vi "HardWare_Phsical Channels Config_Gantner.vi"() -> ()   [LabVIEW 2016]
uses:
  ToolKit/Popup/Public/PSPOP_Popup Cluster.ctl
  ToolKit/Popup/Private/Ctrls/PSPOP_Grid.Cell Info.ctl
  ToolKit/Popup/Private/Ctrls/POP_Data Type.ctl
  HardWare/Ctrls/HardWare _ Data Queue Manage FGV Operation.ctl
  ToolKit/Toolbar/net/SubVIs/TBA_NET_Item.ctl
  HardWare/Ctrls/HardWare Gen _ DAQ Queue Names FGV Operations.ctl
  HardWare/Gantner/DAQ FGV Operations.ctl
  Architecture/Queue Management/ARC_Queue Create_Single.vi
  Architecture/Queue Management/ARC_Queue Remove Element.vi
  Architecture/Queue Management/ARC_Queue Valid.vi
  Architecture/Queue Management/ARC_Queue Insert Element.vi
  Architecture/Queue Management/ARC_Queue Destroy_Single.vi
panel:
  in  "Popups":T1 {"Time" format="%<%Y/%m/%d %I:%M:%S>T"; "Boolean" items=["False", "True"]; "Ring" items=["False", "True"]}
  in  "Cell Info (type only)":T2={"Tag"="", "Row"=0, "Column"=0, "In Symbol?"=FALSE, "In Data?"=FALSE, "Cell String"="", "Ctl Refnum"=refnum, "Prop Type"=enum."Unkown", "Ring Strings"=[], "Ring Values"=[], "New Cell String"=""}
  in  "Tree":string(tree)
  out "Current State":string
  in  "Parameter":cluster{"Q-Local":string, "Variant":variant}
  # "/* -------- Notes for All Users -------- */\nRecommand : \n[1].Display Setting Resolution -> 1440x900\n[2].Read Arch Notes First.\n[3].Make A Call When You Are In Trouble.\n\nTeam Members:\nPansino Soft,Pansino SDMA\n\nCopyright@2013 Pansino.Beijing\n\nVersion Number: 2013"
  # "Boolean Colors"
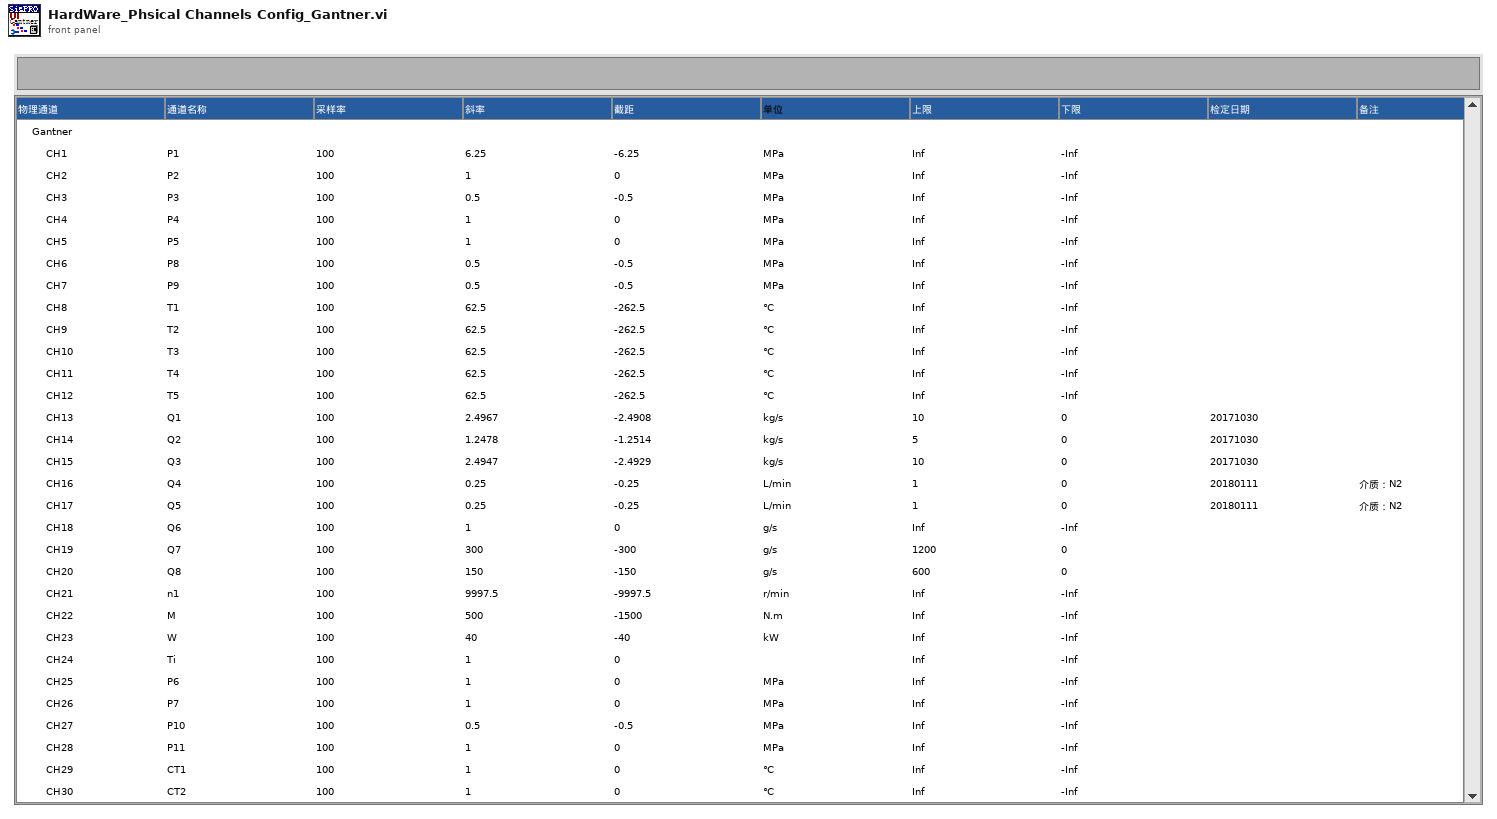
[diagram p1: front panel]
types:
  T1 = typedef "PSPOP_Popup Cluster.ctl" = cluster{"Unknown":bool, "Unknown 2":bool, "String":string, "Integer":i32, "Float":dbl, "Color":u32, "Boolean":u32, "Ring":u32, "Captioned String":cluster{"String":string, "OK":bool, "Cancel":bool}, "Captioned Integer":cluster{"First":i32, "OK":bool, "Cancel":bool}, "Boolean Colors":cluster{"False":cluster{"FG":u32, "BG":u32}, "True":cluster{"FG":u32, "BG":u32}, "T  to  F":cluster{"FG":u32, "BG":u32}, "F  to  T":cluster{"FG":u32, "BG":u32}, "OK":bool, "Cancel":bool}, "2-Int Cluster":cluster{"First":i32, "Second":i32, "OK":bool, "Cancel":bool}, "4-Int Cluster":cluster{"First":i32, "Second":i32, "Third":i32, "Fourth":i32, "OK":bool, "Cancel":bool}, "6-Dbl Cluster":cluster{"First":dbl, "Second":dbl, "Third":dbl, "Fourth":dbl, "Fourth 2":dbl, "Third 2":dbl, "OK":bool, "Cancel":bool}, "Path":path, "Combox":string, "Time":timestamp, "ShortCut":string}
  T2 = typedef "PSPOP_Grid.Cell Info.ctl" = cluster{"Tag":string, "Row":i32, "Column":i32, "In Symbol?":bool, "In Data?":bool, "Cell String":string, "Ctl Refnum":refnum<vi>, "Prop Type":T3, "Ring Strings":string[], "Ring Values":ext[], "New Cell String":string}
  T3 = typedef "POP_Data Type.ctl" = enum16{"NO POPUP", "Unkown", "String", "Integer", "Float", "Color", "Boolean", "Ring", "Captioned String", "Captioned Integer", "Button Color", "2 Int Cluster", "4 Int Cluster", "6-Dbl Cluster", "Path", "Combox", "Time", "ShotCut String"}
  T4 = cluster{"LocalName":string, "System Config":path, "DynaThreads":path, "DataBuf":refnum<queue>, "VIRef":refnum<vi>}
  T5 = typedef "HardWare _ Channel Configurations PopUp Type.ctl" = cluster{"Pop Type":T3, "PopValue":string}
  T6 = cluster{"Error":errorcluster, "Ref":cluster{"VIRef":refnum<vi>, "Tree":refnum<vi>, "CallerVI":refnum<vi>}, "Exit":bool, " Paths":cluster{"PathInActive":path, "ModCfg":path, "CHdef":path, "DT folder":path}, "Q-Local":cluster{"Q-Local Name":string, "Q-Local Order":string, "Q-Local Data":variant}, "Q-HighLevel":cluster{"Q-HighLevel Name":string, "Q-HighLevel Order":string, "Q-HighLevel Data":variant}, "Q-DAQ":cluster{"Q-LowLevel Name[]":string[], "Q-LowLevel Order":string, "Q-LowLevel Data":variant}, "PopUp":string, "Chan Para":cluster{"ParaNames":string[], "DfltValues":string[], "Types":string[], "PopTypes":T5[]}, "Q_DAQs[]":string[], "ActiveModu":cluster{"Tag":string, "CHtype":string}, "ColInfo":cluster{"ColName[]":string[], "ColAlias[]":string[], "ColLength[]":i32[]}, "UsedChList[]":cluster{"ModuTag":string, "ModuAlias":string, "ChanTag[]":string[], "ChanAlias[]":string[], "ChanUnit[]":string[]}[], "DataBuf":refnum<queue>, "Units[]":string[], "ColHeaders[]":string[]}
  T7 = typedef "HardWare _ Data Queue Manage FGV Operation.ctl" = enum16{"Initialize", "Add", "Read", "All"}
  T8 = typedef "TBA_NET_Item.ctl" = cluster{"Tag":string, "Name":string, "Tip":string, "Image":path, "DisplayStyle":i32, "Enable":bool, "Visible":bool}
  T9 = cluster{"Status":string[], "Item":cluster{"Item":T8[]}[]}
  T10 = typedef "HardWare Gen _ DAQ Queue Names FGV Operations.ctl" = enum16{"Initialize", "AddName", "ReadName"}
  T11 = cluster{"Column":i32, "Row":i32, "Formula":string}
  T12 = typedef "DAQ FGV Operations.ctl" = enum16{"Search", "ReadCFG", "ReadVCH", "UpdateTempCFG", "DownloadCFG", "OpenCFG", "ImportPara", "Config", "Start", "Read", "Stop", "Clear"}
  T13 = cluster{"ParaNames":string[], "DfltValues":string[], "Types":string[], "PopTypes":T5[]}
  T14 = cluster{"Q-Local Name":string, "输出簇 2":cluster{"Status":string[], "Item":cluster{"Item":T8[]}[]}}
  T15 = cluster{"Q-Local Name":string, "DataBuf":refnum<queue>}
  T16 = cluster{"ModuTag":string, "ModuAlias":string, "ChanTag[]":string[], "ChanAlias[]":string[], "ChanUnit[]":string[]}[]
  T17 = cluster{"ParaNames":string[], "DfltPara":string[], "Types":string[], "PopTypes":T5[]}
  T18 = cluster{"ColName[]":string[], "ColAlias[]":string[], "ColLength[]":i32[]}
  T19 = typedef "HardWare _ Module Configuration.ctl" = cluster{"ModuName":string, "ModuAlias":string, "ModuSN":string, "CHtype":string, "ParaNames[]":string[], "Paravalues[]":string[][]}
  T20 = cluster{"SlopeA":string, "InterceptB":string, "Unit":string, "AlarmMax":string, "AlarmMin":string, "CheckTime":string, "Note":string, "ChanName":string, "SensorNo.":string}[]
  T21 = typedef "LVPoint32TypeDef.ctl" = cluster{"Horizontal":i32, "Vertical":i32}
  T22 = typedef "POP_Popup Call Parameters.ctl" = cluster{"Prop Type":T3, "Initial Value":variant, "Caption Strings":string[], "Ring Strings":string[], "Cell Rect":cluster{"left":i16, "top":i16, "right":i16, "bottom":i16}, "Mouse Coords":cluster{"x":i16, "y":i16}, "Call Data":variant, "Ring Values":ext[], "Browse Options":T23, "Combo Box":cluster{"Allow Undefined Strings":bool}}
  T23 = typedef "LVBrowseOptionsTypeDef.ctl" = cluster{"Prompt":string, "Match Pattern":string, "Mode":enum32{"existing file", "new file", "new or existing file", "existing dir", "new dir", "new or existing dir", "existing file (use LLBs)", "new file (use LLBs)", "new or existing file (use LLBs)", "new or existing file or directory (use LLBs)", "existing dir (use LLBs)", "new dir (use LLBs)", "new or existing dir (use LLBs)", "existing file or dir", "new file or dir", "new or existing file or dir", "existing file or dir (use LLBs)", "new file or dir (use LLBs)"}, "Start Path":path, "Pattern Label":string, "Button Text":string}
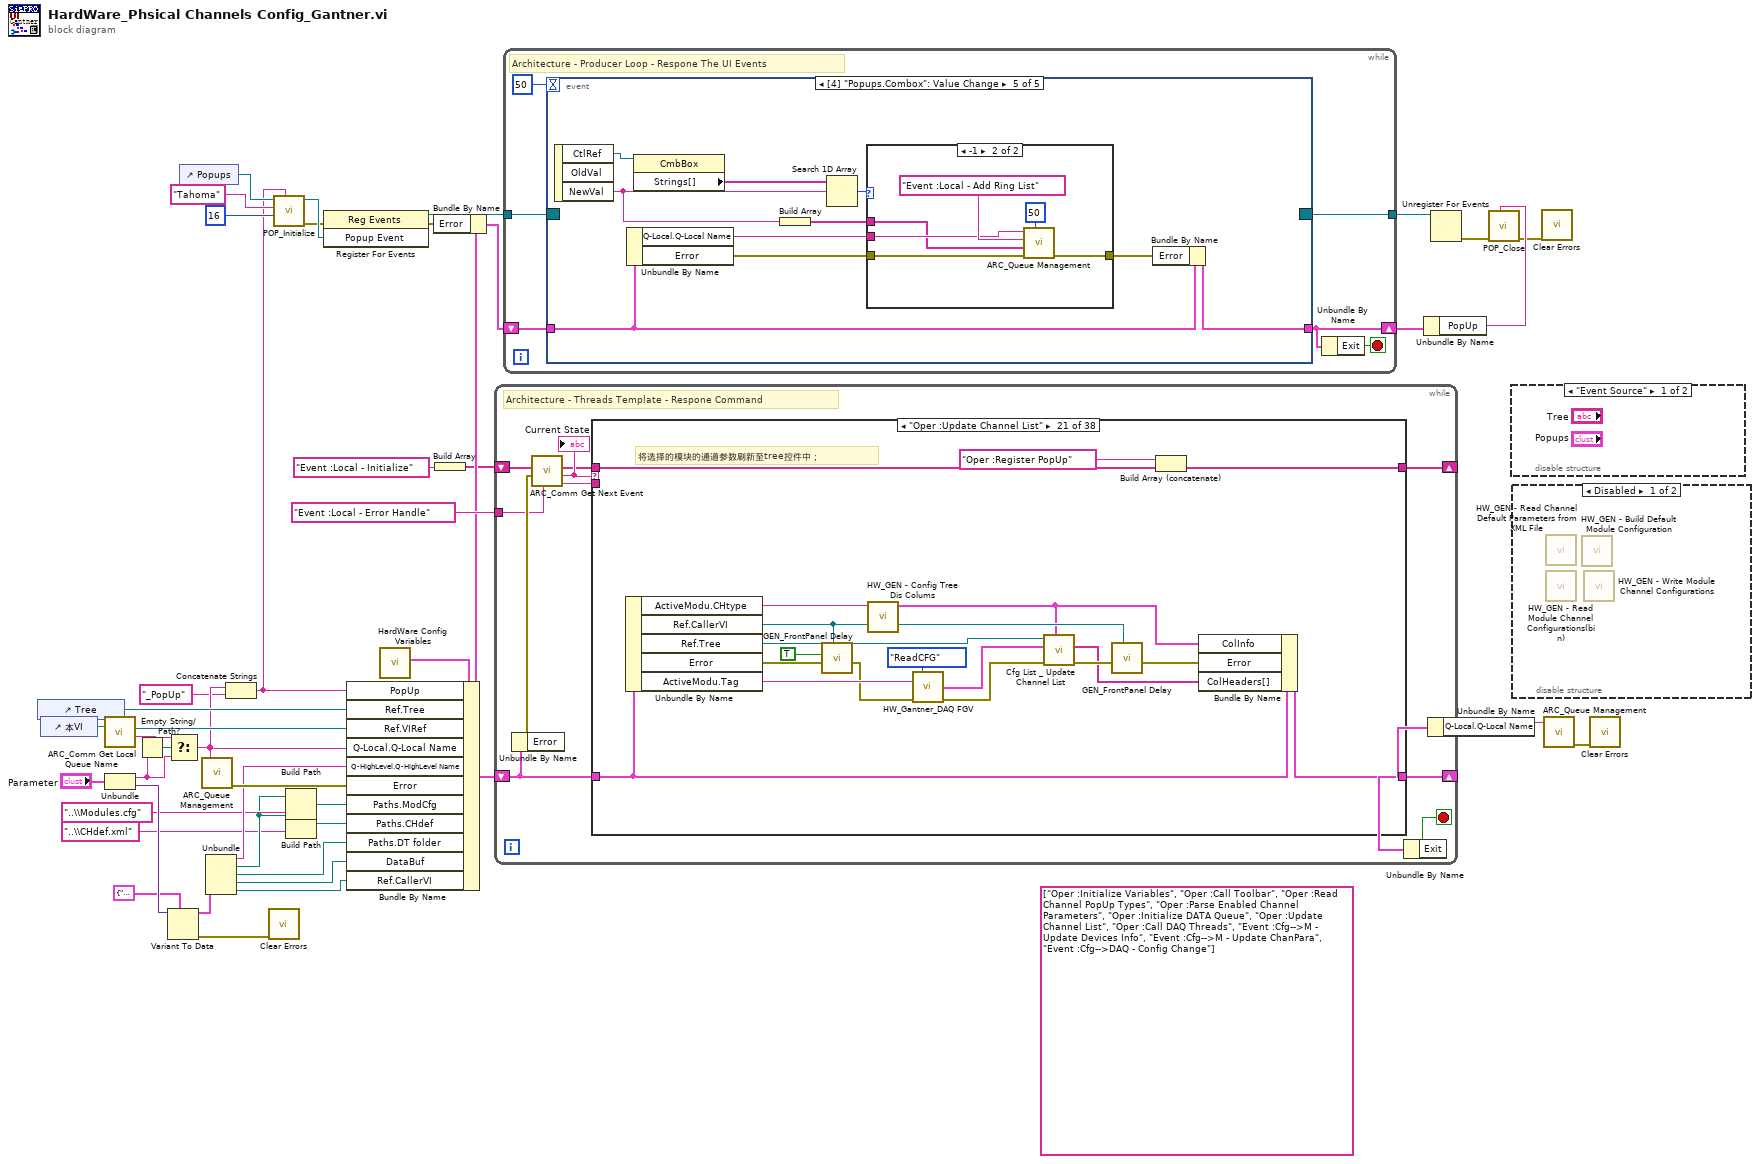
[diagram p0: block diagram]
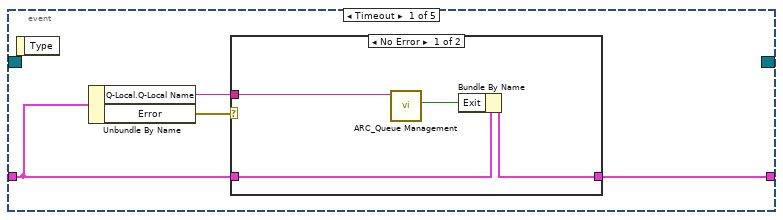
[diagram p3: hidden frame]
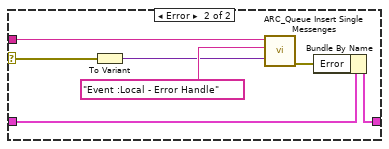
[diagram p4: hidden frame]
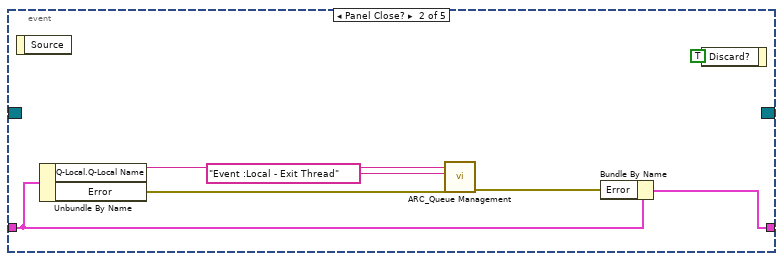
[diagram p5: hidden frame]
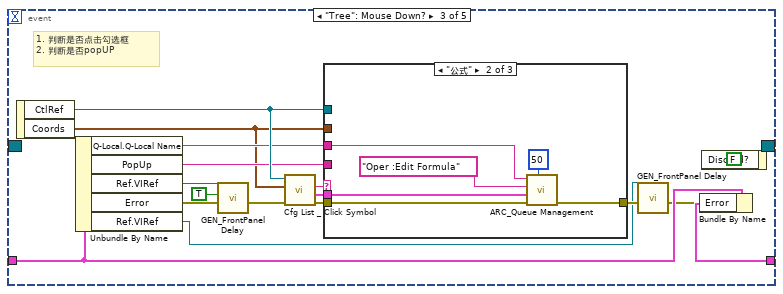
[diagram p6: hidden frame]
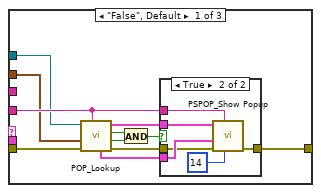
[diagram p7: hidden frame]
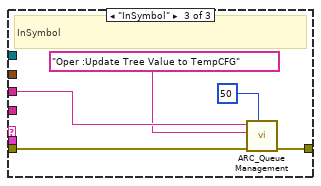
[diagram p9: hidden frame]
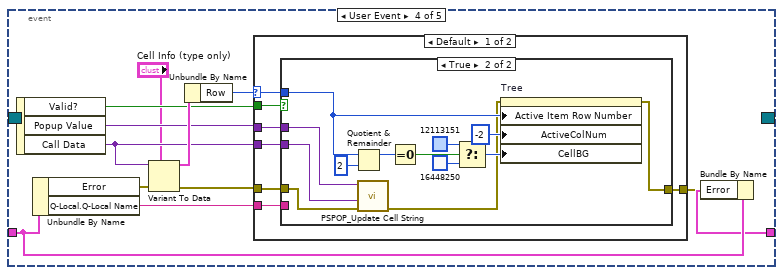
[diagram p10: hidden frame]
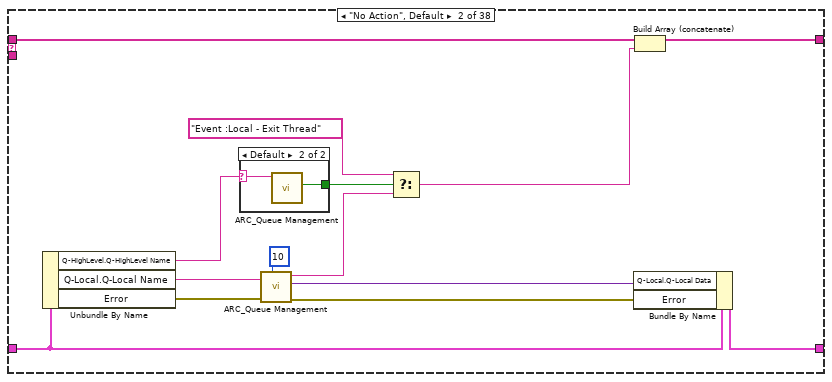
[diagram p16: hidden frame]
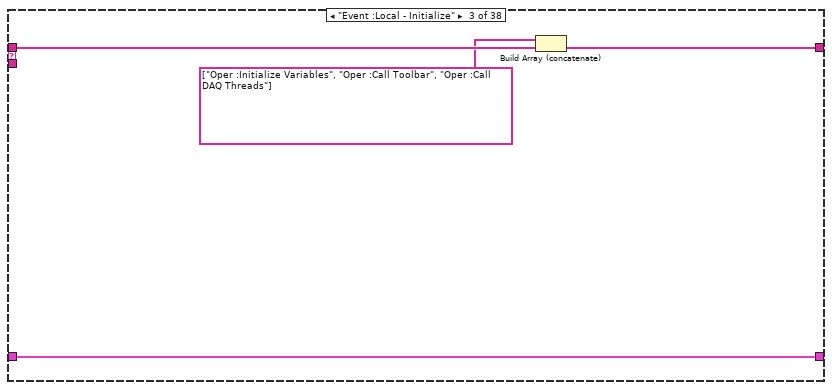
[diagram p18: hidden frame]
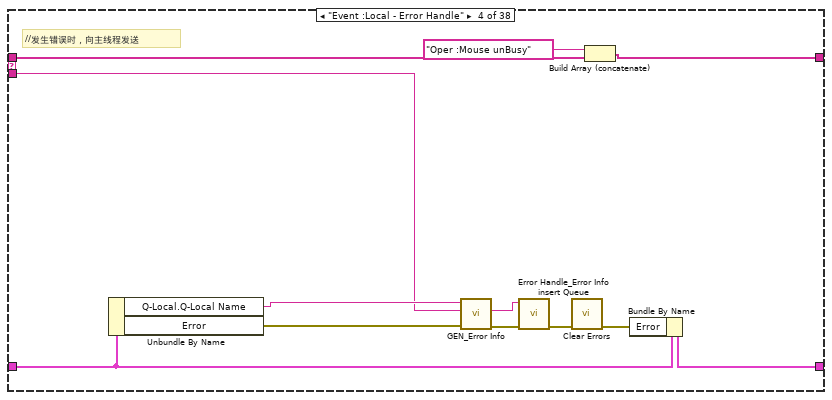
[diagram p19: hidden frame]
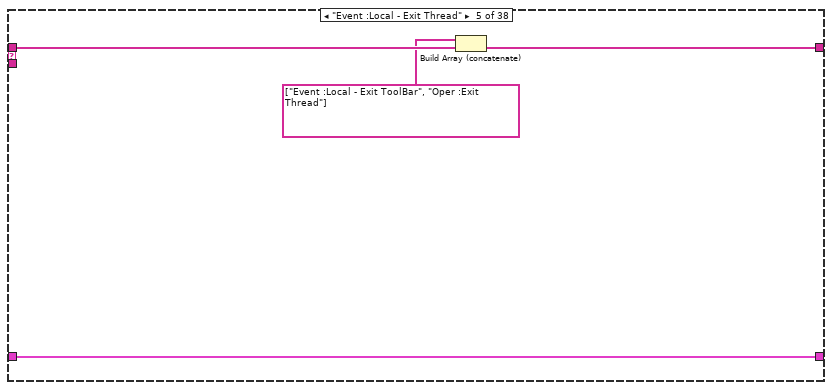
[diagram p20: hidden frame]
diagram:
  (unwired) string[] ["Oper :Initialize Variables", "Oper :Call Toolbar", "Oper :Read Channel PopUp Types", "Oper :Parse Enabled Channel Parameters", "Oper :Initialize DATA Queue", "Oper :Update Channel List", "Oper :Call DAQ Threads", "Event :Cfg-->M - Update Devices Info", "Event :Cfg-->M - Update ChanPara", "Event :Cfg-->DAQ - Config Change"] ("数组")
  n1 = control-ref of="Tree"() -> (w28:refnum<vi>)
  n2 = control-ref of="本VI"() -> (w30:refnum<vi>)
  n3 = call "ARC_Comm Get Local Queue Name.vi"("VI Ref"=w30) -> ("VI  Name"=w31:string, "VI Ref out"=w29:refnum<vi>)  [unwired: 8 in, 1 out]
  n4 = Unbundle("Parameter") -> ("Q-Local"=w33:string, "Variant"=w43:variant)
  n5 = Empty String/Path?(string/path=w33) -> (empty?=w34:bool)
  n6 = Variant To Data(type=T4 {"LocalName"="", "System Config"=path "", "DynaThreads"=path "", "DataBuf"=refnum, "VIRef"=refnum} ("output cluster"), Variant=w43) -> (data=w44:T4, error out=w35:errorcluster)  [unwired: 1 in]
  n7 = Select(t=w31, s=w34, f=w33) -> (s? t:f=w22:string)
  n8 = control-ref of="Popups"() -> (w27:refnum<vi>)
  n9 = call-poly "ARC_Queue Management.vi"("Queue Name"=w22) -> ("error out"=w45:errorcluster)  [unwired: 8 in, 2 out]
  n10 = Unbundle(w44) -> ("LocalName"=w11:string, "System Config"=w6:path, "DynaThreads"=w10:path, "DataBuf"=w3:refnum<queue>, "VIRef"=w1:refnum<vi>)
  n11 = Concatenate Strings(w22, "_PopUp" ("字符串")) -> (w12:string)
  n12 = call <vilib>:"Clear Errors.vi"("error in (no error)"=w35) -> ()  [unwired: 5 in, 2 out]
  n13 = call "POP_Initialize.vi"("Name"=w12, "Font Size"=u32 16, "TontName"="Tahoma", "Popup Cluster Ref"=w27) -> ("error out"=w23:errorcluster, "Popup Event"=w24:refnum<user-event>)  [unwired: 6 in]
  n14 = Build Path(base path=w6, name or relative path="..\\Modules.cfg" ("名称或相对路径")) -> (appended path=w9:path)
  n15 = Build Path(base path=w6, name or relative path="..\\CHdef.xml" ("名称或相对路径")) -> (appended path=w7:path)
  n16 = register-events(error in=w23, w24) -> (reference out=w20:refnum<event-registration>, error out=w18:errorcluster)  [unwired: 1 in]
  n17 = call "HardWare Config Variables.vi"() -> ("HardWare_Phsical Channels Config.vi"=w32:T6)  [unwired: 11 in]
  n18 = Bundle By Name(cluster=w32, "PopUp"=w12, "Ref.Tree"=w28, "Ref.VIRef"=w29, "Q-Local.Q-Local Name"=w22, "Q-HighLevel.Q-HighLevel Name"=w11, "Error"=w45, "Paths.ModCfg"=w9, "Paths.CHdef"=w7, "Paths.DT folder"=w10, "DataBuf"=w3, "Ref.CallerVI"=w1) -> (w38:T6)
  n19 = Bundle By Name(cluster=w38, "Error"=w18) -> (w19:T6)
  n20 = Build Array("Event :Local - Initialize") -> (w36:string[])
  n21 = while {
    shift-right: [w49] -> w41
    shift-left: w38 -> [w51]
    shift-right: [w52] -> _
    shift-left: w36 -> [w55]
    tunnel: "Event :Local - Error Handle" ("Error Handle") -> [w47]
    stop <- w48 stop-if-true
    # "Architecture - Threads Template - Respone Command"
    n22 = Unbundle By Name(w51) -> ("Error"=w50:errorcluster)
    n23 = call "ARC_Comm Get Next Event.vi"("Error Handle"=w47, "error in (no error)"=w50, "event queue in"=w55) -> ("prev event"=w46:string, "next event"=w54:string, "event queue out"=w53:string[])  [unwired: 3 in]
    "Current State" <- w54
    n24 = case shown="\"Oper :Update Channel List\"" w54 {
      selector: w54 -> [_ _ _ _ _ _ _ _ _ _ _ _ _ _ _ _ _ _ _ _ _ _ _ _ _ _ _ _ _ _ _ _ w420 w426 w432 _ _ _]
      tunnel: w51 -> [w56 w71 w76 w87 w90 w100 w107 w111 w123 w134 w154 w178 w181 w201 w213 w217 w220 w225 w229 w236 w256 w261 w271 w280 w284 w303 w316 w332 w367 w402 w413 w416 w419 w425 w431 w437 w444 w459]
      tunnel: w53 -> [w57 w69 w77 w89 w93 w101 w104 w112 w124 w135 w155 w179 w197 w200 w210 w218 w223 w228 w230 w238 w257 w269 w273 w281 w283 w288 w317 w337 w363 w403 w415 w417 w424 w430 w436 w438 w447 w462]
      tunnel: [w57 w68 w75 w85 w92 w98 w109 w112 w124 w135 w153 w177 w197 w199 w209 w215 w223 w228 w230 w238 w248 w269 w272 w281 w285 w287 w315 w337 w362 w390 w414 w417 w423 w429 w435 w438 w447 w462] -> w52
      tunnel: [w56 w70 w76 w88 w90 w99 w110 w111 w120 w133 w142 w176 w180 w201 w212 w216 w220 w225 w229 w234 w253 w260 w270 w280 w284 w292 w316 w331 w366 w392 w413 w416 w421 w427 w433 w437 w443 w458] -> w49
      tunnel: w46 -> [_ _ _ w79 _ _ _ _ _ _ _ _ _ _ _ _ _ _ _ _ _ _ _ _ _ _ _ _ _ w395 _ _ _ _ _ _ _ _]
      frame "----------Core Status----------" {
      }
      frame "No Action", Default {
        n25 = Unbundle By Name(w71) -> ("Q-HighLevel.Q-HighLevel Name"=w63:string, "Q-Local.Q-Local Name"=w64:string, "Error"=w65:errorcluster)
        n26 = case shown="Default" w63 {
          selector: w63 -> [_ w72]
          tunnel: [_ w73] -> w61
          frame "" {
          }
          frame Default {
            n27 = call-poly "ARC_Queue Management.vi"("Queue Name(unamed)"=w72) -> ("Not Exist?"=w73:bool)  [unwired: 8 in, 2 out]
          }
        }
        n28 = call-poly "ARC_Queue Management.vi"("Time out(-1)_queue out"=10, "error in (no error)"=w65, "Queue Name(unamed)"=w64) -> ("error out"=w67:errorcluster, "Data"=w66:variant, "Event"=w59:string)  [unwired: 5 in, 1 out]
        n29 = Select(t="Event :Local - Exit Thread" ("Event"), s=w61, f=w59) -> (s? t:f=w58:string)
        n30 = Bundle By Name(cluster=w71, "Q-Local.Q-Local Data"=w66, "Error"=w67) -> (w70:T6)
        n31 = Build Array (concatenate)(w69, w58) -> (w68:string[])
      }
      frame "Event :Local - Initialize" {
        n32 = Build Array (concatenate)(string[] ["Oper :Initialize Variables", "Oper :Call Toolbar", "Oper :Call DAQ Threads"] ("数组"), w77) -> (w75:string[])
      }
      frame "Event :Local - Error Handle" {
        # "//发生错误时，向主线程发送"
        n33 = Unbundle By Name(w87) -> ("Q-Local.Q-Local Name"=w80:string, "Error"=w81:errorcluster)
        n34 = call "GEN_Error Info.vi"("error in"=w81, "Event name"=w79, "Thread name"=w80) -> ("error out"=w84:errorcluster, "Error Report"=w83:string)  [unwired: 7 in]
        n35 = call "Error Handle_Error Info insert Queue.vi"("error in"=w84, "error info in"=w83) -> ("error out"=w82:errorcluster)  [unwired: 9 in]
        n36 = call <vilib>:"Clear Errors.vi"("error in (no error)"=w82) -> ("error out"=w86:errorcluster)  [unwired: 5 in, 1 out]
        n37 = Build Array (concatenate)("Oper :Mouse unBusy", w89) -> (w85:string[])
        n38 = Bundle By Name(cluster=w87, "Error"=w86) -> (w88:T6)
      }
      frame "Event :Local - Exit Thread" {
        n39 = Build Array (concatenate)(string[] ["Event :Local - Exit ToolBar", "Oper :Exit Thread"] ("数组"), w93) -> (w92:string[])
      }
      frame "Event :Local - Exit ToolBar" {
        n40 = Build Array("PhyChanTBA" ("Q-LowLevel.Q-LowLevel Name")) -> (w94:string[])
        n41 = Bundle By Name(cluster=w100, "Q-DAQ.Q-LowLevel Name[]"=w94, "Q-DAQ.Q-LowLevel Order"="UI :L_Evnt - Exit" ("Q-LowLevel.Q-LowLevel Order")) -> (w99:T6)
        n42 = Build Array (concatenate)(string[] ["Oper :Send To LowLevel"] ("数组"), w101) -> (w98:string[])
      }
      frame "Event :Local - Add Ring List" {
        n43 = Unbundle By Name(w107) -> ("Q-Local.Q-Local Data"=w105:variant, "Error"=w106:errorcluster)
        n44 = Variant To Data(error in=w106, type=w104, Variant=w105) -> (data=w103:string[], error out=w102:errorcluster)
        n45 = Build Array (concatenate)(string[] ["Oper :Add Ring List", "Oper :Register PopUp"] ("数组"), w104) -> (w109:string[])
        n46 = Bundle By Name(cluster=w107, "Units[]"=w103, "Error"=w102) -> (w110:T6)
      }
      frame "----------Operations----------" {
      }
      frame "Oper :Initialize Variables" {
        n47 = Unbundle By Name(w123) -> ("Ref.Tree"=w119:refnum<vi>, "Ref.VIRef"=w121:refnum<vi>, "Error"=w122:errorcluster, "Paths.ModCfg"=w117:path)
        n48 = call "GEN_FrontPanel Delay.vi"("VI ref"=w121, "错误输入（无错误）"=w122) -> ("错误输出"=w118:errorcluster)  [unwired: 9 in]
        n49 = call "TREE_Clear.vi"("error in"=w118, "Tree Ref"=w119) -> ("error out"=w116:errorcluster)  [unwired: 8 in, 1 out]
        n50 = call "HW_GEN - Data Queue Manage FGV.vi"("Oper."=HardWare___Data_Queue_Manage_FGV_Operation."Initialize", "error in"=w116) -> ("error out"=w115:errorcluster)  [unwired: 7 in, 2 out]
        n51 = Bundle By Name(cluster=w123, "Error"=w115, "Paths.PathInActive"=w117, "ActiveModu.Tag"="" ("ActiveModTag")) -> (w120:T6)
      }
      frame "Oper :Register PopUp" {
        # "//读取文件中对通道配置参数的类型定义\n定义每一列PopUp的类型"
        n52 = Unbundle By Name(w134) -> ("PopUp"=w130:string, "Ref.Tree"=w131:refnum<vi>, "Chan Para"=w126:T13, "ColHeaders[]"=w128:string[], "Error"=w129:errorcluster)
        n53 = call "Cfg List _ Index Col PopUp Types.vi"("error in"=w129, "ColHeaders[]"=w128, "Chan Para"=w126) -> ("error out"=w125:errorcluster, "ColPopupTypes[]"=w127:T5[])  [unwired: 7 in]
        n54 = call "Cfg PopUp _ Registration.vi"("PopUp"=w130, "error in"=w125, "ColTypes[ ]"=w127, "Ref.Tree"=w131) -> ("error out"=w132:errorcluster)  [unwired: 7 in]
        n55 = Bundle By Name(cluster=w134, "Error"=w132) -> (w133:T6)
      }
      frame "Oper :Call Toolbar" {
        # "//\n1、动态调用Toolbar UI.vi\n2、将其插入子面板中"
        n56 = Unbundle By Name(w154) -> ("Error"=w151:errorcluster, "Q-Local.Q-Local Name"=w138:string)
        n57 = vi-ref "Toobar UI.vi"() -> (w152:refnum<vi>)
        n58 = property class="VI"(reference=w152, error in=w151) -> (error out=w149:errorcluster, "Path"=w150:path)  [unwired: 1 out]
        n59 = Bundle("Q-Local Name"=w138, "输出簇 2"=T9 {"Status"=["Init", "Download", "Open", "Save", "Save As", "ImportPara"], "Item"=[{"Item"=[{"Tag"="Download", "Name"="下载", "Tip"="下载配置", "Image"=path "", "DisplayStyle"=3, "Enable"=TRUE, "Visible"=TRUE}, {"Tag"="Open", "Name"="打开", "Tip"="打开配置文件", "Image"=path "", "DisplayStyle"=3, "Enable"=TRUE, "Visible"=TRUE}, {"Tag"="Save", "Name"="保存", "Tip"="保存配置参数", "Image"=path "", "DisplayStyle"=3, "Enable"=TRUE, "Visible"=TRUE}, {"Tag"="Save As", "Name"="另存为", "Tip"="参数另存为", "Image"=path "", "DisplayStyle"=3, "Enable"=TRUE, "Visible"=TRUE}, {"Tag"="ImportPara", "Name"="导入参数", "Tip"="读取参数文件", "Image"=path "", "DisplayStyle"=3, "Enable"=TRUE, "Visible"=TRUE}]}, {"Item"=[{"Tag"="Download", "Name"="下载", "Tip"="下载配置", "Image"=path "", "DisplayStyle"=3, "Enable"=TRUE, "Visible"=TRUE}, {"Tag"="Open", "Name"="打开", "Tip"="打开配置文件", "Image"=path "", "DisplayStyle"=3, "Enable"=TRUE, "Visible"=TRUE}, {"Tag"="Save", "Name"="保存", "Tip"="保存配置参数", "Image"=path "", "DisplayStyle"=3, "Enable"=TRUE, "Visible"=TRUE}, {"Tag"="Save As", "Name"="另存为", "Tip"="参数另存为", "Image"=path "", "DisplayStyle"=3, "Enable"=TRUE, "Visible"=TRUE}, {"Tag"="ImportPara", "Name"="导入参数", "Tip"="读取参数文件", "Image"=path "", "DisplayStyle"=3, "Enable"=TRUE, "Visible"=TRUE}]}, {"Item"=[{"Tag"="Download", "Name"="下载", "Tip"="下载配置", "Image"=path "", "DisplayStyle"=3, "Enable"=TRUE, "Visible"=TRUE}, {"Tag"="Open", "Name"="打开", "Tip"="打开配置文件", "Image"=path "", "DisplayStyle"=3, "Enable"=TRUE, "Visible"=TRUE}, {"Tag"="Save", "Name"="保存", "Tip"="保存配置参数", "Image"=path "", "DisplayStyle"=3, "Enable"=TRUE, "Visible"=TRUE}, {"Tag"="Save As", "Name"="另存为", "Tip"="参数另存为", "Image"=path "", "DisplayStyle"=3, "Enable"=TRUE, "Visible"=TRUE}, {"Tag"="ImportPara", "Name"="导入参数", "Tip"="读取参数文件", "Image"=path "", "DisplayStyle"=3, "Enable"=TRUE, "Visible"=TRUE}]}, {"Item"=[{"Tag"="Download", "Name"="下载", "Tip"="下载配置", "Image"=path "", "DisplayStyle"=3, "Enable"=TRUE, "Visible"=TRUE}, {"Tag"="Open", "Name"="打开", "Tip"="打开配置文件", "Image"=path "", "DisplayStyle"=3, "Enable"=TRUE, "Visible"=TRUE}, {"Tag"="Save", "Name"="保存", "Tip"="保存配置参数", "Image"=path "", "DisplayStyle"=3, "Enable"=TRUE, "Visible"=TRUE}, {"Tag"="Save As", "Name"="另存为", "Tip"="参数另存为", "Image"=path "", "DisplayStyle"=3, "Enable"=TRUE, "Visible"=TRUE}, {"Tag"="ImportPara", "Name"="导入参数", "Tip"="读取参数文件", "Image"=path "", "DisplayStyle"=3, "Enable"=TRUE, "Visible"=TRUE}]}, {"Item"=[{"Tag"="Download", "Name"="下载", "Tip"="下载配置", "Image"=path "", "DisplayStyle"=3, "Enable"=TRUE, "Visible"=TRUE}, {"Tag"="Open", "Name"="打开", "Tip"="打开配置文件", "Image"=path "", "DisplayStyle"=3, "Enable"=TRUE, "Visible"=TRUE}, {"Tag"="Save", "Name"="保存", "Tip"="保存配置参数", "Image"=path "", "DisplayStyle"=3, "Enable"=TRUE, "Visible"=TRUE}, {"Tag"="Save As", "Name"="另存为", "Tip"="参数另存为", "Image"=path "", "DisplayStyle"=3, "Enable"=TRUE, "Visible"=TRUE}, {"Tag"="ImportPara", "Name"="导入参数", "Tip"="读取参数文件", "Image"=path "", "DisplayStyle"=3, "Enable"=TRUE, "Visible"=TRUE}]}]}) -> (w137:T14)  [unwired: 1 in]
        n60 = call "ARC_Dynamic Call_Reentrant.vi"("command queue name"="PhyChanTBA", "open front panel? (T)"=FALSE, "error in (no error)"=w149, "parameter else"=w137, "control name"="Parameter", "vi path"=w150) -> ("error out"=w146:errorcluster, "time out"=w144:bool, "call failed"=w145:bool, "VI Ref"=w140:refnum<vi>)  [unwired: 2 in]
        n61 = Or(x=w145, y=w144) -> (x .or. y?=w143:bool)
        n62 = case shown="False" w143 {
          tunnel: w146 -> [w158 w159]
          tunnel: [w157 w159] -> w141
          tunnel: w140 -> [w156 _]
          frame False {
            n63 = invoke on="Toolbar Subpanel" class="SubPnl" method="Insert VI"(error in=w158, "VI Ref"=w156) -> (error out=w157:errorcluster)  [unwired: 2 in, 3 out]
          }
          frame True {
          }
        }
        n64 = Build Array (concatenate)(w155) -> (w153:string[])
        n65 = Bundle By Name(cluster=w154, "Error"=w141) -> (w142:T6)
      }
      frame "Oper :Call DAQ Threads" {
        # "根据配置文件内容中的DeviceName调用相应的DAQ线程"
        n66 = Unbundle By Name(w178) -> ("Error"=w172:errorcluster, "Q-Local.Q-Local Name"=w168:string, "DataBuf"=w160:refnum<queue>)
        n67 = vi-ref "DAQ Thread_Gantner.vi"() -> (w173:refnum<vi>)
        n68 = property class="VI"(reference=w173, error in=w172) -> (error out=w171:errorcluster, "Path"=w170:path, "Name"=w166:string)  [unwired: 1 out]
        n69 = Match Pattern(string=w166, regular expression=".vi") -> (before substring=w162:string)  [unwired: 1 in, 3 out]
        n70 = Build Array (concatenate)(w179) -> (w177:string[])
        n71 = Bundle("Q-Local Name"=w168, "DataBuf"=w160) -> (w169:T15)  [unwired: 1 in]
        n72 = call "ARC_Dynamic Call_Single.vi"("command queue name"=w162, "open front panel? (T)"=FALSE, "error in (no error)"=w171, "parameter else"=w169, "control name"="Parameter", "vi path"=w170) -> ("error out"=w165:errorcluster)  [unwired: 3 in, 2 out]
        n73 = Build Array(w162) -> (w161:string[])
        n74 = call "HW_GEN - DAQ Queue Names Management.vi"("Oper."=HardWare_Gen___DAQ_Queue_Names_FGV_Operations."AddName", "error in"=w165, "Qname in"=w162) -> ("error out"=w164:errorcluster)  [unwired: 7 in, 1 out]
        n75 = Bundle By Name(cluster=w178, "Error"=w164, "Q-DAQ.Q-LowLevel Name[]"=w161) -> (w176:T6)
      }
      frame "Oper :Edit Formula" {
        # "编辑公式界面；\n根据当前界面中选择的物理通道刷新虚拟通道界面中的channel list"
        n76 = Unbundle By Name(w181) -> ("Ref.Tree"=w187:refnum<vi>, "Q-Local.Q-Local Data"=w182:variant, "Error"=w183:errorcluster, "UsedChList[]"=w196:T16)
        n77 = Variant To Data(error in=w183, type=T11 {"Column"=0, "Row"=0, "Formula"=""} ("Cluster"), Variant=w182) -> (data=w185:T11, error out=w184:errorcluster)
        n78 = Unbundle By Name(w185) -> ("Column"=w188:i32, "Row"=w189:i32, "Formula"=w195:string)
        n79 = call "PSVCH_Formula Edit.vi"("error in"=w184, "UsedChList[]"=w196, "Formula In"=w195) -> ("Error Out"=w190:errorcluster, "Formula"=w193:string, "Cancel?"=w192:bool)  [unwired: 6 in]
        n80 = Select(t=w195, s=w192, f=w193) -> (s? t:f=w194:string)
        n81 = property class="Tree (strict)"(reference=w187, error in=w190, "ActiveColNum"=w188, "Active Item Row Number"=w189, "Cell String"=w194) -> (error out=w191:errorcluster)  [unwired: 1 out]
        n82 = Bundle By Name(cluster=w181, "Error"=w191) -> (w180:T6)
      }
      frame "Oper :Refresh SelectCH" {
        # "选择通道后，更新临时配置信息，刷新虚拟通道中的通道列表"
        n83 = Build Array (concatenate)(w200, string[] ["Oper :Update Tree Value to TempCFG"] ("array")) -> (w199:string[])
      }
      frame "Oper :Add Ring List" {
        n84 = Unbundle By Name(w213) -> ("Error"=w203:errorcluster, "Chan Para"=w208:T13, "Units[]"=w202:string[], "Paths.CHdef"=w206:path, "ActiveModu.CHtype"=w205:string)
        n85 = call "HW_GEN - Update Units List.vi"("Units[]"=w202, "Chan dflt Para in"=w208) -> ("Units out"=w204:string, "Chan dflt Para out"=w207:T17)  [unwired: 8 in]
        n86 = call "HW_GEN - Write Channel Default Parameters to XML File.vi"("error in"=w203, "Dflt Units[]"=w204, "ChanType"=w205, "path to XML document"=w206) -> ("错误输出"=w211:errorcluster)  [unwired: 7 in]
        n87 = Bundle By Name(cluster=w213, "Error"=w211, "Chan Para"=w207) -> (w212:T6)
        n88 = Build Array (concatenate)(w210) -> (w209:string[])
      }
      frame "Oper :Exit Thread" {
        n89 = Bundle By Name(cluster=w217, "Exit"=TRUE) -> (w216:T6)
        n90 = Build Array (concatenate)(w218) -> (w215:string[])
      }
      frame "Oper :Mouse Busy" {
        n91 = Unbundle By Name(w220) -> ("Ref.VIRef"=w221:refnum<vi>)
        n92 = call "GEN_FrontPanel Delay.vi"("VI ref"=w221, "delay？"=TRUE) -> ("错误输出"=w219:errorcluster)  [unwired: 9 in]
        n93 = call <vilib>:"Clear Errors.vi"("error in (no error)"=w219) -> ()  [unwired: 5 in, 2 out]
      }
      frame "Oper :Mouse unBusy" {
        n94 = Unbundle By Name(w225) -> ("Ref.VIRef"=w226:refnum<vi>)
        n95 = call "GEN_FrontPanel Delay.vi"("VI ref"=w226, "delay？"=FALSE) -> ("错误输出"=w224:errorcluster)  [unwired: 9 in]
        n96 = call <vilib>:"Clear Errors.vi"("error in (no error)"=w224) -> ()  [unwired: 5 in, 2 out]
      }
      frame "----------Device----------" {
      }
      frame "Oper :Read Channel PopUp Types" {
        n97 = Unbundle By Name(w236) -> ("Paths.CHdef"=w235:path, "ActiveModu.CHtype"=w231:string, "Error"=w237:errorcluster)
        n98 = call "HW_GEN - Read Channel Default Parameters from XML File.vi"("error in"=w237, "ChanType"=w231, "path to XML document"=w235) -> ("错误输出"=w233:errorcluster, "Chan dflt Para out"=w232:T17)  [unwired: 7 in]
        n99 = Bundle By Name(cluster=w236, "Chan Para"=w232, "Error"=w233) -> (w234:T6)
      }
      frame "Oper :Update Channel List" {
        # "将选择的模块的通道参数刷新至tree控件中；"
        n100 = Unbundle By Name(w256) -> ("ActiveModu.CHtype"=w241:string, "Ref.CallerVI"=w249:refnum<vi>, "Ref.Tree"=w254:refnum<vi>, "Error"=w255:errorcluster, "ActiveModu.Tag"=w245:string)
        n101 = call "GEN_FrontPanel Delay.vi"("VI ref"=w249, "错误输入（无错误）"=w255, "delay？"=TRUE) -> ("错误输出"=w244:errorcluster)  [unwired: 8 in]
        n102 = call "HW_GEN - Config Tree Dis Colums.vi"("ActiveModu.CHtype"=w241) -> ("ColInfo"=w240:T18)  [unwired: 10 in]
        n103 = call "HW_Gantner_DAQ FGV.vi"("Oper."=DAQ_FGV_Operations."ReadCFG", "ActiveModuTag"=w245, "error in"=w244) -> ("ActiveCFG"=w242:T19, "error out"=w243:errorcluster)  [unwired: 6 in, 5 out]
        n104 = call "Cfg List _ Update Channel List.vi"("ColInfo"=w240, "错误输入"=w243, "ModuCfg"=w242, "TreeRef"=w254) -> ("错误输出"=w252:errorcluster, "ColHeaders[]"=w239:string[])  [unwired: 6 in]
        n105 = call "GEN_FrontPanel Delay.vi"("VI ref"=w249, "错误输入（无错误）"=w252) -> ("错误输出"=w250:errorcluster)  [unwired: 9 in]
        n106 = Build Array (concatenate)("Oper :Register PopUp", w257) -> (w248:string[])
        n107 = Bundle By Name(cluster=w256, "ColInfo"=w240, "Error"=w250, "ColHeaders[]"=w239) -> (w253:T6)
      }
      frame "Oper :Update Tree Value to TempCFG" {
        # "当前tree控件上对应模块的配置参数更新至临时变量中；\n读取新的ActiveModu的参数信息刷新至tree中。"
        n108 = Unbundle By Name(w261) -> ("Ref.Tree"=w263:refnum<vi>, "Error"=w262:errorcluster, "ColInfo.ColName[]"=w264:string[])
        n109 = call "Cfg List _ Get Current Configurations.vi"("ColInfo.ColName[]"=w264, "error in"=w262, "tree"=w263) -> ("error out"=w267:errorcluster, "TreePara"=w268:cluster{"ColHdrs":string[], "Items":string[][]})  [unwired: 7 in]
        n110 = call "HW_Gantner_DAQ FGV.vi"("Oper."=DAQ_FGV_Operations."UpdateTempCFG", "TreePara"=w268, "error in"=w267) -> ("TempCFG out"=w259:T19[], "error out"=w265:errorcluster)  [unwired: 6 in, 5 out]
        n111 = call "HW_GEN - Select Used Chan List.vi"("Cfg in"=w259) -> ("UsedChList[]"=w258:T16)  [unwired: 9 in, 1 out]
        n112 = Bundle By Name(cluster=w261, "Error"=w265, "UsedChList[]"=w258) -> (w260:T6)
      }
      frame "Oper :Down Load Cfg" {
        # "确认使用当前Tree控件的配置；\n向DAQ线程发送配置信息变化的命令；\n向主线程发送通道信息变化命令；"
        n113 = Unbundle By Name(w271) -> ("Error"=w279:errorcluster)
        n114 = call "HW_Gantner_DAQ FGV.vi"("Oper."=DAQ_FGV_Operations."DownloadCFG", "error in"=w279) -> ("cfg change?"=w276:bool, "error out"=w278:errorcluster)  [unwired: 7 in, 5 out]
        n115 = Build Array (concatenate)(string[] ["Event :Cfg-->DAQ - Config Change", "Event :Cfg-->M - Update ChanPara", "Event :Cfg-->Data - Update Formula Nodes"] ("array"), w273) -> (w277:string[])
        n116 = Select(t=w277, s=w276, f=w273) -> (s? t:f=w272:string[])
        n117 = Bundle By Name(cluster=w271, "Error"=w278) -> (w270:T6)
      }
      frame "----------cmd from other threads-----------" {
      }
      frame "Event :TBA-->Cfg - Download" {
        # "确认使用当前Tree控件的配置；\n1、将当前Tree控件上的信息更新至临时变量中；\n2、下载配置信息；"
        n118 = Build Array (concatenate)(string[] ["Oper :Update Tree Value to TempCFG", "Oper :Down Load Cfg"] ("array"), w283) -> (w285:string[])
      }
      frame "Event :TBA-->Cfg - Open" {
        # "读取配置文件，更新参数变量；\n刷新至tree中"
        n119 = Unbundle By Name(w303) -> ("Paths.PathInActive"=w289:path, "Paths.ModCfg"=w301:path, "Error"=w302:errorcluster)
        n120 = call "文件对话框"("start path"=w301, "error in"=w302, "pattern (all files)"="*.cfg", "pattern label"="配置文件" ("pattern (all files)")) -> ("selected path"=w293:path, "exists"=w298:bool, "cancelled"=w297:bool, "error out"=w294:errorcluster)  [unwired: 8 in]
        n121 = Not(x=w297) -> (.not. x?=w296:bool)
        n122 = And(x=w298, y=w296) -> (x .and. y?=w295:bool)
        n123 = case shown="True" w295 {
          tunnel: w294 -> [w305 w310]
          tunnel: w293 -> [_ w308]
          tunnel: [w305 w309] -> w291
          tunnel: [w306 w308] -> w290
          tunnel: w289 -> [w306 _]
          tunnel: w288 -> [w304 w313]
          tunnel: [w304 w312] -> w287
          tunnel: string[] ["Oper :Update Channel List"] ("数组") -> [_ w311]
          frame False {
          }
          frame True {
            n124 = call "HW_Gantner_DAQ FGV.vi"("Oper."=DAQ_FGV_Operations."OpenCFG", "Path.ModuCFG"=w308, "error in"=w310) -> ("error out"=w309:errorcluster)  [unwired: 6 in, 6 out]
            n125 = Build Array (concatenate)(w311, w313) -> (w312:string[])
          }
        }
        n126 = Bundle By Name(cluster=w303, "Paths.PathInActive"=w290, "Error"=w291) -> (w292:T6)
      }
      frame "Event :TBA-->Cfg - Save" {
        # "保存当前配置信息"
        n127 = Build Array (concatenate)(string[] ["Oper :Update Tree Value to TempCFG", "Oper :Down Load Cfg"] ("数组"), w317) -> (w315:string[])
      }
      frame "Event :TBA-->Cfg - Save As" {
        n128 = Unbundle By Name(w332) -> ("Ref.Tree"=w322:refnum<vi>, "ColInfo.ColName[]"=w323:string[], "Paths.PathInActive"=w330:path, "Paths.ModCfg"=w335:path, "Error"=w336:errorcluster)
        n129 = Get Date/Time String() -> (date string=w328:string, time string=w327:string)  [unwired: 3 in]
        n130 = Concatenate Strings(w328, "_" ("字符串"), w327, ".cfg" ("字符串")) -> (w324:string)
        n131 = call "文件对话框2"("start path"=w335, "default name"=w324, "error in"=w336, "pattern (all files)"="*.cfg", "pattern label"="配置文件" ("pattern (all files)")) -> ("selected path"=w329:path, "cancelled"=w320:bool, "error out"=w321:errorcluster)  [unwired: 7 in, 1 out]
        n132 = Select(t=w330, s=w320, f=w329) -> (s? t:f=w319:path)
        n133 = case shown="False" w320 {
          tunnel: w323 -> [w345 _]
          tunnel: w322 -> [w344 _]
          tunnel: w321 -> [w343 w348]
          tunnel: w319 -> [w340 _]
          tunnel: [w339 w348] -> w318
          frame False {
            n134 = call "Cfg List _ Get Current Configurations.vi"("ColInfo.ColName[]"=w345, "error in"=w343, "tree"=w344) -> ("error out"=w346:errorcluster, "TreePara"=w347:cluster{"ColHdrs":string[], "Items":string[][]})  [unwired: 7 in]
            n135 = call "HW_Gantner_DAQ FGV.vi"("Oper."=DAQ_FGV_Operations."UpdateTempCFG", "TreePara"=w347, "error in"=w346) -> ("TempCFG out"=w338:T19[], "error out"=w341:errorcluster)  [unwired: 6 in, 5 out]
            n136 = call "HW_GEN - Write Module Channel Configurations(bin).vi"("error in"=w341, "ModuCfg"=w338, "Path"=w340) -> ("error out"=w339:errorcluster)  [unwired: 8 in]
          }
          frame True {
          }
        }
        n137 = Bundle By Name(cluster=w332, "Error"=w318) -> (w331:T6)
      }
      frame "Event :TBA-->Cfg - ImportPara" {
        n138 = Unbundle By Name(w367) -> ("Ref.CallerVI"=w349:refnum<vi>, "Ref.VIRef"=w354:refnum<vi>, "Error"=w357:errorcluster, "Chan Para"=w361:T13)
        n139 = call "GEN_FrontPanel Delay.vi"("VI ref"=w354, "错误输入（无错误）"=w357, "delay？"=TRUE) -> ("错误输出"=w353:errorcluster)  [unwired: 8 in]
        n140 = call <vilib>:"Set Busy.vi"("error in (no error)"=w353, "VI reference (current VI)"=w349) -> ("error out"=w352:errorcluster)  [unwired: 8 in, 1 out]
        n141 = call "ParaExcel _ Read.vi"("error in"=w352) -> ("error out"=w365:errorcluster, "Units[]"=w359:string[], "data out"=w364:T20)  [unwired: 8 in]
        n142 = case shown="No Error" w365 {
          selector: w365 -> [w381 w386]
          tunnel: [w374 w384] -> w356
          tunnel: w364 -> [w376 _]
          tunnel: w363 -> [w379 w383]
          tunnel: [w378 w383] -> w362
          tunnel: w361 -> [w375 w382]
          tunnel: [w375 w382] -> w360
          frame No Error {
            # "从excel文件中加载新的参数\n将加载的单位加入下拉列表中"
            n143 = call "HW_Gantner_DAQ FGV.vi"("Oper."=DAQ_FGV_Operations."ImportPara", "error in"=w381, "ImportPara"=w376) -> ("error out"=w374:errorcluster)  [unwired: 6 in, 6 out]
            n144 = Build Array (concatenate)(string[] ["Oper :Update Channel List", "Oper :Add Ring List"] ("数组"), w379) -> (w378:string[])
          }
          frame Error {
            n145 = call <vilib>:"Simple Error Handler.vi"("error in (no error)"=w386) -> ("error out"=w385:errorcluster)  [unwired: 4 in, 4 out]
            n146 = call <vilib>:"Clear Errors.vi"("error in (no error)"=w385) -> ("error out"=w384:errorcluster)  [unwired: 5 in, 1 out]
          }
        }
        n147 = flat-sequence {
          tunnel: w356 -> [w371]
          tunnel: w354 -> [w369]
          tunnel: [w370] -> w351
          tunnel: [w368] -> w350
          tunnel: w349 -> [w368]
          tunnel: [w373] -> w355
          tunnel: w351 -> [w373]
          tunnel: w350 -> [w372]
          frame #0 {
            n148 = call "GEN_FrontPanel Delay.vi"("VI ref"=w369, "错误输入（无错误）"=w371) -> ("错误输出"=w370:errorcluster)  [unwired: 9 in]
          }
          frame #1 {
            n149 = call <vilib>:"Unset Busy.vi"("VI reference (current VI)"=w372) -> ()  [unwired: 10 in, 1 out]
          }
        }
        n150 = Bundle By Name(cluster=w367, "Error"=w355, "Chan Para"=w360, "Units[]"=w359) -> (w366:T6)
      }
      frame "Event :Main-->Cfg - Module Change" {
        # "当前tree控件上对应模块的配置参数更新至临时变量中；\n读取新的ActiveModu的参数信息刷新至tree中。"
        n151 = Unbundle By Name(w402) -> ("Ref.Tree"=w399:refnum<vi>, "ActiveModu.Tag"=w400:string, "Error"=w401:errorcluster, "ColInfo.ColName[]"=w398:string[], "Q-Local.Q-Local Data"=w396:variant)
        n152 = case shown="Default" w400 {
          tunnel: w401 -> [w408 w411]
          tunnel: [w405 w411] -> w397
          tunnel: w399 -> [w409 _]
          tunnel: w398 -> [w407 _]
          frame Default {
            n153 = call "Cfg List _ Get Current Configurations.vi"("ColInfo.ColName[]"=w407, "error in"=w408, "tree"=w409) -> ("error out"=w406:errorcluster, "TreePara"=w404:cluster{"ColHdrs":string[], "Items":string[][]})  [unwired: 7 in]
            n154 = call "HW_Gantner_DAQ FGV.vi"("Oper."=DAQ_FGV_Operations."UpdateTempCFG", "TreePara"=w404, "error in"=w406) -> ("error out"=w405:errorcluster)  [unwired: 6 in, 6 out]
          }
          frame "" {
          }
        }
        n155 = Variant To Data(error in=w397, type=w395, Variant=w396) -> (data=w387:string, error out=w394:errorcluster)
        n156 = call "HW_Gantner_DAQ FGV.vi"("Oper."=DAQ_FGV_Operations."ReadCFG", "ActiveModuTag"=w387, "error in"=w394) -> ("ActiveModuCHtype"=w388:string, "error out"=w391:errorcluster)  [unwired: 6 in, 5 out]
        n157 = Bundle By Name(cluster=w402, "ActiveModu.CHtype"=w388, "Error"=w391, "ActiveModu.Tag"=w387) -> (w392:T6)
        n158 = Build Array (concatenate)(string[] ["Oper :Read Channel PopUp Types", "Oper :Update Channel List", "Event :Cfg-->M - Unbusy Mouse"] ("array"), w403) -> (w390:string[])
      }
      frame "Event :Main-->Cfg - Start DAQ" {
        # "主线程在搜索完硬件后向该线程发送启动DAQ命令；\n启动DAQ线程；\n下载当前配置；"
        n159 = Build Array (concatenate)(string[] ["Event :TBA-->Cfg - Download", "Event :Main-->Cfg - Module Change", "Event :Cfg-->DAQ - Config Change", "Event :Cfg-->M - Update ChanPara"] ("event queue out"), w415) -> (w414:string[])
      }
      frame "------------send to other threads----------" {
      }
      frame "Event :Cfg-->M - Update ChanPara" {
        # "//向显示线程发送硬件配置"
        n160 = Unbundle By Name(w419) -> ("UsedChList[]"=w418:T16)
        n161 = Bundle By Name(cluster=w419, "Q-HighLevel.Q-HighLevel Order"=w420, "Q-HighLevel.Q-HighLevel Data"=w418) -> (w421:T6)
        n162 = Build Array (concatenate)("Oper :Send To HighLevel" ("Error Handle"), w424) -> (w423:string[])
      }
      frame "Event :Cfg-->M - Unbusy Mouse" {
        # "//向显示线程发送硬件配置"
        n163 = Bundle By Name(cluster=w425, "Q-HighLevel.Q-HighLevel Order"=w426) -> (w427:T6)
        n164 = Build Array (concatenate)("Oper :Send To HighLevel" ("Error Handle"), w430) -> (w429:string[])
      }
      frame "Event :Cfg-->DAQ - Config Change" {
        # "//配置参数发生改变，将新的参数发送至DAQ线程"
        n165 = Bundle By Name(cluster=w431, "Q-DAQ.Q-LowLevel Order"=w432) -> (w433:T6)
        n166 = Build Array (concatenate)("Oper :Send To LowLevel" ("Error Handle"), w436) -> (w435:string[])
      }
      frame "----------Communication----------" {
      }
      frame "Oper :Send To HighLevel" {
        n167 = Unbundle By Name(w444) -> ("Q-HighLevel.Q-HighLevel Name"=w446:string, "Q-HighLevel.Q-HighLevel Order"=w441:string, "Q-HighLevel.Q-HighLevel Data"=w440:variant, "Error"=w445:errorcluster)
        n168 = call-poly "ARC_Queue Management.vi"("Queue Name(unamed)"=w446) -> ("Not Exist?"=w442:bool)  [unwired: 8 in, 2 out]
        n169 = case shown="False" w442 {
          tunnel: w445 -> [w453 w454]
          tunnel: w446 -> [w451 _]
          tunnel: w441 -> [w449 _]
          tunnel: w440 -> [w450 _]
          tunnel: [w448 w454] -> w439
          frame False {
            n170 = call-poly "ARC_Queue Management.vi"("Time out(-1)_queue in"=50, "error in (no error)"=w453, "Data"=w450, "Event"=w449, "Queue Name(unamed)"=w451) -> ("error out"=w448:errorcluster)  [unwired: 5 in, 1 out]
          }
          frame True {
          }
        }
        n171 = Bundle By Name(cluster=w444, "Error"=w439) -> (w443:T6)
      }
      frame "Oper :Send To LowLevel" {
        # ">> Notes: 如不具备底层线程，可删除此分支；\n如具备多个底层线程，可修改为队列的数组。<<"
        n172 = Unbundle By Name(w459) -> ("Q-DAQ.Q-LowLevel Name[]"=w461:string[], "Q-DAQ.Q-LowLevel Order"=w457:string, "Q-DAQ.Q-LowLevel Data"=w456:variant, "Error"=w460:errorcluster)
        n173 = for {
          tunnel: w461 -> [w468] mode=indexing
          tunnel: w457 -> [w465]
          tunnel: w456 -> [w464]
          shift-right: [w463] -> w455
          shift-left: w460 -> [w467]
          n174 = call-poly "ARC_Queue Management.vi"("Queue Name(unamed)"=w468) -> ("Not Exist?"=w466:bool)  [unwired: 8 in, 2 out]
          n175 = case shown="False" w466 {
            tunnel: w467 -> [w474 w475]
            tunnel: w468 -> [w472 _]
            tunnel: w465 -> [w470 _]
            tunnel: w464 -> [w471 _]
            tunnel: [w469 w475] -> w463
            frame False {
              n176 = call-poly "ARC_Queue Management.vi"("Time out(-1)_queue in"=50, "error in (no error)"=w474, "Data"=w471, "Event"=w470, "Queue Name(unamed)"=w472) -> ("error out"=w469:errorcluster)  [unwired: 5 in, 1 out]
            }
            frame True {
            }
          }
        }
        n177 = Bundle By Name(cluster=w459, "Error"=w455) -> (w458:T6)
      }
    }
    n178 = Unbundle By Name(w49) -> ("Exit"=w48:bool)
  }
  n179 = while {
    shift-right: [w479] -> w15
    shift-left: w19 -> [w480]
    tunnel: w20 -> [w477]
    tunnel: [w476] -> w17
    stop <- w478 stop-if-true
    # "Architecture - Producer Loop - Respone The UI Events"
    n180 = event shown="[4] \"Popups.Combox\": Value Change" {
      selector: w477 -> [_ _ _ _ _]
      dyn-events: [_ _ _ _ _] -> w476
      timeout: 50 -> [_ _ _ _ _]
      tunnel: w480 -> [w484 w501 w520 w553 w592]
      tunnel: [w485 w500 w519 w552 w589] -> w479
      event Timeout {
        n181 = event-data() -> ()  [unwired: 1 in, 1 out]
        n182 = Unbundle By Name(w484) -> ("Q-Local.Q-Local Name"=w483:string, "Error"=w482:errorcluster)
        n183 = case shown="No Error" w482 {
          selector: w482 -> [_ w496]
          tunnel: [w489 w494] -> w485
          tunnel: w484 -> [w487 w495]
          tunnel: w483 -> [w486 w493]
          frame No Error {
            n184 = call-poly "ARC_Queue Management.vi"("Queue Name(unamed)"=w486) -> ("Not Exist?"=w488:bool)  [unwired: 8 in, 2 out]
            n185 = Bundle By Name(cluster=w487, "Exit"=w488) -> (w489:T6)
          }
          frame Error {
            n186 = To Variant(anything=w496) -> (Variant=w491:variant)
            n187 = call "ARC_Queue Insert Single Messenges.vi"("Data"=w491, "Order"="Event :Local - Error Handle" ("Event"), "Queue Name"=w493) -> ("error out"=w490:errorcluster)  [unwired: 8 in]
            n188 = Bundle By Name(cluster=w495, "Error"=w490) -> (w494:T6)
          }
        }
      }
      event Panel Close? {
        n189 = event-data() -> ()  [unwired: 1 in, 1 out]
        n190 = Unbundle By Name(w501) -> ("Q-Local.Q-Local Name"=w498:string, "Error"=w502:errorcluster)
        n191 = call-poly "ARC_Queue Management.vi"("error in (no error)"=w502, "Event"="Event :Local - Exit Thread", "Queue Name(unamed)"=w498) -> ("error out"=w499:errorcluster)  [unwired: 7 in, 1 out]
        n192 = Bundle By Name(cluster=w501, "Error"=w499) -> (w500:T6)
        n193 = event-data("Discard?"=TRUE ("放弃？")) -> ()  [unwired: 1 in, 1 out]
      }
      event "Tree": Mouse Down? {
        # "1. 判断是否点击勾选框\n2. 判断是否popUP"
        n194 = event-data() -> ("CtlRef"=w518:refnum<vi>, "Coords"=w504:T21)  [unwired: 1 in]
        n195 = Unbundle By Name(w520) -> ("Q-Local.Q-Local Name"=w507:string, "PopUp"=w509:string, "Ref.VIRef"=w510:refnum<vi>, "Error"=w516:errorcluster, "Ref.VIRef"=w508:refnum<vi>)
        n196 = call "GEN_FrontPanel Delay.vi"("VI ref"=w510, "错误输入（无错误）"=w516, "delay？"=TRUE ("Delay?")) -> ("错误输出"=w515:errorcluster)  [unwired: 8 in]
        n197 = call "Cfg List _ Click Symbol.vi"("错误输入"=w515, "坐标"=w504, "TreeRef"=w518) -> ("错误输出"=w517:errorcluster, "Cluster"=w505:T11, "Click Colum"=w506:string)  [unwired: 6 in]
        n198 = case shown="\"公式\"" w506 {
          tunnel: w509 -> [w531 _ _]
          tunnel: [w524 w541 w548] -> w512
          tunnel: w518 -> [w523 _ _]
          tunnel: w517 -> [w522 w542 w549]
          tunnel: w507 -> [_ w539 w547]
          tunnel: w505 -> [_ w540 _]
          tunnel: w504 -> [w521 _ _]
          frame "False", Default {
            n199 = call "POP_Lookup.vi"("Name"=w531, "error in (no error)"=w522, "Point"=w521, "Ctl Refnum"=w523) -> ("error out"=w530:errorcluster, "In Bounds?"=w526:bool, "Found"=w525:bool, "Popup Parameters"=w528:T22, "Cell Info (Call data)"=w529:T2)  [unwired: 3 in]
            n200 = And(x=w525, y=w526) -> (x .and. y?=w527:bool)
            n201 = case shown="True" w527 {
              tunnel: w528 -> [_ w538]
              tunnel: w529 -> [_ w537]
              tunnel: w530 -> [w532 w536]
              tunnel: w531 -> [_ w535]
              tunnel: [w532 w534] -> w524
              frame False {
              }
              frame True {
                n202 = call "PSPOP_Show Popup.vi"("Font Size"=u32 14, "Name"=w535, "error in (no error)"=w536, "Call Data (ignore if empty)"=w537, "Popup Parameters"=w538) -> ("error out"=w534:errorcluster)  [unwired: 6 in]
              }
            }
          }
          frame "公式" {
            n203 = call-poly "ARC_Queue Management.vi"("Time out(-1)_queue in"=50, "error in (no error)"=w542, "Data"=w540, "Event"="Oper :Edit Formula" ("Queue Name(unamed)"), "Queue Name(unamed)"=w539) -> ("error out"=w541:errorcluster)  [unwired: 5 in, 1 out]
          }
          frame "InSymbol" {
            # "InSymbol"
            n204 = call-poly "ARC_Queue Management.vi"("Time out(-1)_queue in"=50, "error in (no error)"=w549, "Event"="Oper :Update Tree Value to TempCFG", "Queue Name(unamed)"=w547) -> ("error out"=w548:errorcluster)  [unwired: 6 in, 1 out]
          }
        }
        n205 = call "GEN_FrontPanel Delay.vi"("VI ref"=w508, "错误输入（无错误）"=w512) -> ("错误输出"=w513:errorcluster)  [unwired: 9 in]
        n206 = Bundle By Name(cluster=w520, "Error"=w513) -> (w519:T6)
        n207 = event-data("Discard?"=FALSE ("放弃？")) -> ()  [unwired: 1 in, 1 out]
      }
      event User Event {
        n208 = event-data() -> ("Valid?"=w559:bool, "Popup Value"=w556:variant, "Call Data"=w557:variant)  [unwired: 1 in]
        n209 = Unbundle By Name(w553) -> ("Error"=w558:errorcluster, "Q-Local.Q-Local Name"=w550:string)
        n210 = Variant To Data(error in=w558, type="Cell Info (type only)", Variant=w557) -> (data=w560:T2, error out=w561:errorcluster)
        n211 = Unbundle By Name(w560) -> ("Row"=w554:i32)
        n212 = case shown="Default" w554 {
          selector: w554 -> [w562 _]
          tunnel: w559 -> [w568 _]
          tunnel: w556 -> [w567 _]
          tunnel: w557 -> [w566 _]
          tunnel: w561 -> [w565 w583]
          tunnel: [w564 w583] -> w551
          tunnel: w550 -> [w563 _]
          frame Default {
            n213 = case shown="True" w568 {
              tunnel: w567 -> [_ w581]
              tunnel: w566 -> [_ w582]
              tunnel: w565 -> [w569 w580]
              tunnel: [w569 w570] -> w564
              tunnel: w563 -> [_ _]
              tunnel: w562 -> [_ w572]
              frame False {
              }
              frame True {
                n214 = Quotient & Remainder(x=w572, y=2) -> (x-y*floor(x/y)=w578:i32)  [unwired: 1 out]
                n215 = call "PSPOP_Update Cell String.vi"("error in (no error)"=w580, "Call Data (must be Cell Info cluster)"=w582, "Popup Value"=w581) -> ("error out"=w571:errorcluster)  [unwired: 7 in, 1 out]
                n216 = Equal To 0?(x=w578) -> (x = 0?=w577:bool)
                n217 = Select(t=u32 12113151, s=w577, f=u32 16448250) -> (s? t:f=w573:u32)
                n218 = property on="Tree" class="Tree (严格)"(error in=w571, "Active Item Row Number"=w572, "ActiveColNum"=-2 ("Active Cell:Active Column Number"), "CellBG"=w573) -> (error out=w570:errorcluster)  [unwired: 1 in, 1 out]
              }
            }
          }
          frame -1 {
          }
        }
        n219 = Bundle By Name(cluster=w553, "Error"=w551) -> (w552:T6)
      }
      event Value Change {
        n220 = event-data() -> ("CtlRef"=w593:refnum<vi>, "NewVal"=w585:string)  [unwired: 1 in, 1 out]
        n221 = Unbundle By Name(w592) -> ("Q-Local.Q-Local Name"=w591:string, "Error"=w590:errorcluster)
        n222 = property class="CmbBox"(reference=w593) -> ("Strings[]"=w586:string[])  [unwired: 1 in, 2 out]
        n223 = Build Array(w585) -> (w584:string[])
        n224 = Search 1D Array(1D array=w586, element=w585) -> (index of element=w587:i32)  [unwired: 1 in]
        n225 = case shown="-1" w587 {
          tunnel: w591 -> [_ w598]
          tunnel: w590 -> [w594 w597]
          tunnel: [w594 w596] -> w588
          tunnel: w584 -> [_ w595]
          frame 0, Default {
          }
          frame -1 {
            n226 = call-poly "ARC_Queue Management.vi"("Time out(-1)_queue in"=50, "error in (no error)"=w597, "Data"=w595, "Event"="Event :Local - Add Ring List" ("Queue Name(unamed)"), "Queue Name(unamed)"=w598) -> ("error out"=w596:errorcluster)  [unwired: 5 in, 1 out]
          }
        }
        n227 = Bundle By Name(cluster=w592, "Error"=w588) -> (w589:T6)
      }
    }
    n228 = Unbundle By Name(w479) -> ("Exit"=w478:bool)
  }
  n229 = Unbundle By Name(w15) -> ("PopUp"=w14:string)
  n230 = Unbundle By Name(w41) -> ("Q-Local.Q-Local Name"=w40:string)
  n231 = Unregister For Events(event registration refnum=w17) -> (error out=w16:errorcluster)  [unwired: 1 in]
  n232 = call "POP_Close.vi"("Name"=w14, "error in (no error)"=w16) -> ("error out"=w13:errorcluster)  [unwired: 9 in]
  n233 = disable-structure shown="\"Event Source\"" {
    frame condition #0 (active) {
    }
    frame condition #1 {
    }
  }
  n234 = disable-structure shown="Disabled" {
    frame Disabled {
      n235 = call "HW_GEN - Read Channel Default Parameters from XML File.vi"() -> ()  [unwired: 10 in, 2 out]
      n236 = call "HW_GEN - Read Module Channel Configurations(bin).vi"() -> ()  [unwired: 10 in, 2 out]
      n237 = call "HW_GEN - Build Default Module Configuration.vi"() -> ()  [unwired: 10 in, 2 out]
      n238 = call "HW_GEN - Write Module Channel Configurations.vi"() -> ()  [unwired: 11 in, 1 out]
    }
    frame Enabled {
    }
  }
  n239 = call <vilib>:"Clear Errors.vi"("error in (no error)"=w13) -> ()  [unwired: 5 in, 2 out]
  n240 = call-poly "ARC_Queue Management.vi"("Queue Name(unamed)"=w40) -> ("error out"=w4:errorcluster)  [unwired: 8 in, 2 out]
  n241 = call <vilib>:"Clear Errors.vi"("error in (no error)"=w4) -> ()  [unwired: 5 in, 2 out]
